vi "Convert Num to Farrads.vi"(1 "String":string) -> (0 "Numeric":dbl)   [LabVIEW 2013]
panel:
  out "Numeric (SI Notation)":dbl format="%#_6p"
  # "µ"
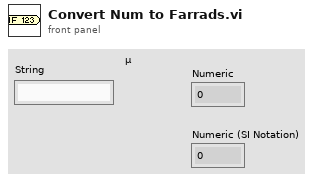
[diagram p1: front panel]
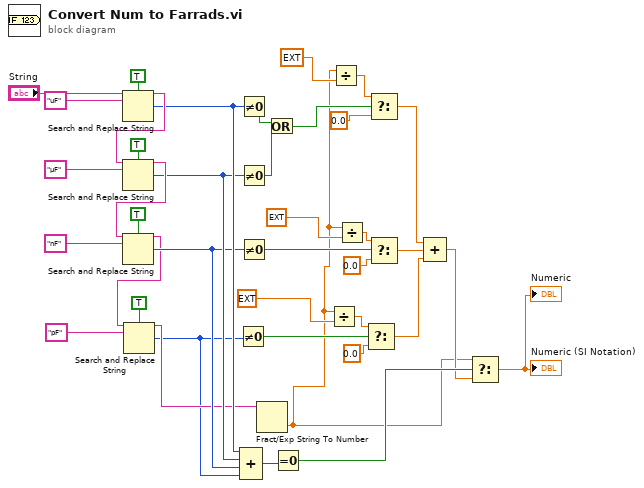
[diagram p0: block diagram]
diagram:
  n1 = Search and Replace String(case sensitive?=TRUE ("ignore case? (F)"), input string="String", search string="uF") -> (result string=w34:string, number of replacements=w21:i32)  [unwired: 5 in, 2 out]
  n2 = Search and Replace String(case sensitive?=TRUE ("ignore case? (F)"), input string=w34, search string="µF") -> (result string=w31:string, number of replacements=w20:i32)  [unwired: 5 in, 2 out]
  n3 = Search and Replace String(case sensitive?=TRUE ("ignore case? (F)"), input string=w31, search string="nF") -> (result string=w9:string, number of replacements=w19:i32)  [unwired: 5 in, 2 out]
  n4 = Search and Replace String(case sensitive?=TRUE ("ignore case? (F)"), input string=w9, search string="pF") -> (result string=w8:string, number of replacements=w1:i32)  [unwired: 5 in, 2 out]
  n5 = Not Equal To 0?(x=w1) -> (x != 0?=w7:bool)
  n6 = Not Equal To 0?(x=w21) -> (x != 0?=w14:bool)
  n7 = Not Equal To 0?(x=w20) -> (x != 0?=w13:bool)
  n8 = Not Equal To 0?(x=w19) -> (x != 0?=w30:bool)
  n9 = Compound Arithmetic op=ADD(w21, w20, w19, w1) -> (w18:i32)
  n10 = Fract/Exp String To Number(string=w8) -> (number=w2:dbl)  [unwired: 3 in, 1 out]
  n11 = Or(x=w14, y=w13) -> (x .or. y?=w12:bool)
  n12 = Equal To 0?(x=w18) -> (x = 0?=w17:bool)
  n13 = Divide(x=w2, y=ext 1000000000000.0) -> (x/y=w4:ext)
  n14 = Divide(x=w2, y=ext 1000000.0) -> (x/y=w29:ext)
  n15 = Divide(x=w2, y=ext 1000000000.0) -> (x/y=w25:ext)
  n16 = Select(t=w4, s=w7, f=0.0) -> (s? t:f=w3:ext)
  n17 = Select(t=w29, s=w12, f=0.0) -> (s? t:f=w23:ext)
  n18 = Select(t=w25, s=w30, f=0.0) -> (s? t:f=w24:ext)
  n19 = Compound Arithmetic op=ADD(w23, w24, w3) -> (w16:ext)
  n20 = Select(t=w2, s=w17, f=w16) -> (s? t:f=→"Numeric" →"Numeric (SI Notation)":ext)
